vi "Load config.vi"(8 "error in (no error)":errorcluster, 11 "Data Cluster in":T1) -> (0 "error out":errorcluster, 2 "Call config dialog?":bool, 3 "Data Cluster out":T1)   [LabVIEW 2020, in "UI.lvlib"]
uses:
  UI.lvlib
  Module Data--cluster.ctl
  <vilib>/Utility/file.llb/Application Directory.vi
  <vilib>/Utility/config.llb/Read Key (String).vi
  <vilib>/Utility/config.llb/Read Key (Double).vi
  <vilib>/Utility/config.llb/NI_LVConfig.lvlib
  NI_DAQ/Libraries/NI DAQ/NI DAQ.lvlib
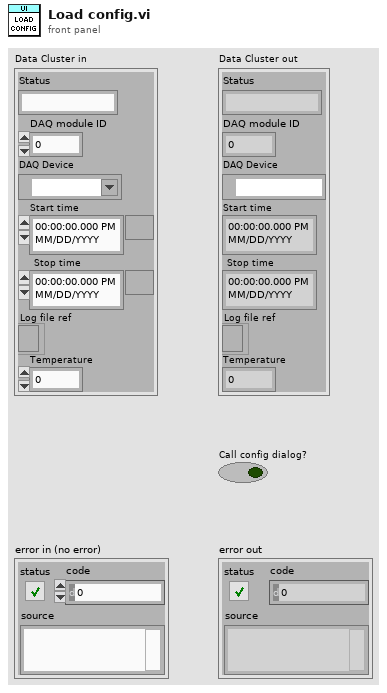
[diagram p1: front panel]
types:
  T1 = typedef "UI.lvlib/Module Data--cluster.ctl" = cluster{"Status":string, "DAQ module ID":i32, "DAQ Device":tag, "Start time":timestamp, "Stop time":timestamp, "Log file ref":refnum<file>, "Temperature":dbl}
  T2 = typedef "NI_LVConfig.lvlib/Config Data RefNum.ctl" = refnum<k1>
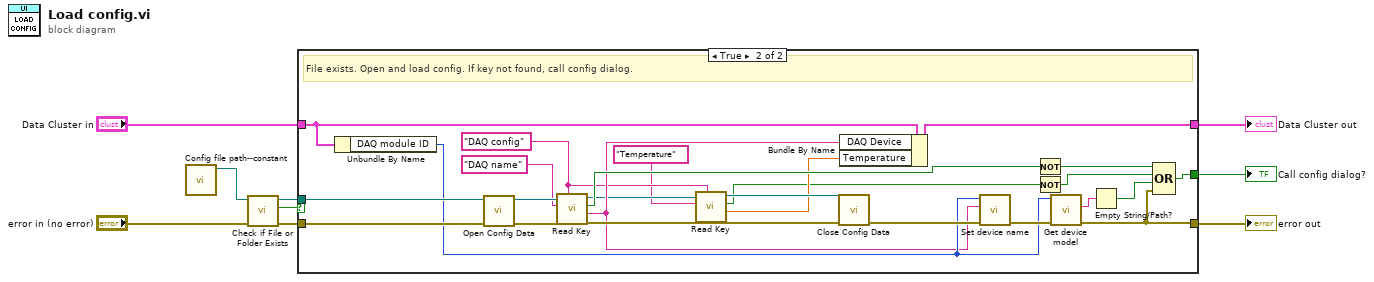
[diagram p0: block diagram]
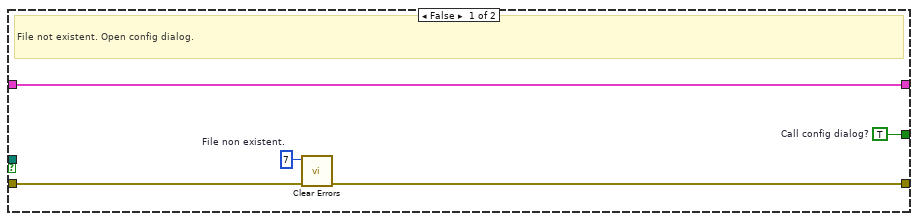
[diagram p2: hidden frame]
diagram:
  n1 = call "Config file path--constant.vi"() -> ("Path"=w3:path)  [unwired: 11 in]
  n2 = call <vilib>:"Check if File or Folder Exists.vi"("error in (no error)"="error in (no error)", "path"=w3) -> ("error out"=w4:errorcluster, "file or folder exists?"=w1:bool, "dup path"=w2:path)  [unwired: 7 in]
  n3 = case shown="True" w1 {
    tunnel: w4 -> [w13 w37]
    tunnel: w2 -> [_ w38]
    tunnel: [w14 w29] -> w9
    tunnel: [w11 w22] -> w6
    tunnel: "Data Cluster in" -> [w12 w30]
    tunnel: [w12 w34] -> w8
    frame False {
      w10 = 7  # File non existent.
      w14 = TRUE  # Call config dialog?
      # "File not existent. Open config dialog."
      n4 = call <vilib>:"Clear Errors.vi"("error in (no error)"=w13, "specific error code to clear (0: all)"=w10) -> ("error out"=w11:errorcluster)  [unwired: 4 in, 1 out]
    }
    frame True {
      w19 = "DAQ config" ("section")
      # "File exists. Open and load config. If key not found, call config dialog."
      n5 = Unbundle By Name(w30) -> ("DAQ module ID"=w24:i32)
      n6 = call <vilib>:"Open Config Data.vi"("error in (no error)"=w37, "configuration file path"=w38) -> ("error out"=w36:errorcluster, "refnum"=w35:T2)  [unwired: 7 in, 1 out]
      n7 = call-poly <vilib>:"Read Key.vi"("section"=w19, "key"="DAQ name", "refnum"=w35) -> ("value"=w23:string, "found?"=w32:bool, "refnum out"=w21:T2)  [unwired: 5 in, 1 out]
      n8 = call-poly <vilib>:"Read Key.vi"("section"=w19, "key"="Temperature", "refnum"=w21) -> ("value"=w17:dbl, "found?"=w16:bool, "refnum out"=w20:T2)  [unwired: 5 in, 1 out]
      n9 = call <vilib>:"Close Config Data.vi"("error in (no error)"=w36, "refnum"=w20) -> ("error out"=w26:errorcluster)  [unwired: 8 in, 1 out]
      n10 = Bundle By Name(cluster=w30, "DAQ Device"=w23, "Temperature"=w17) -> (w34:T1)
      n11 = call "Set device name.vi"("error in"=w26, "Device name"=w23, "Module ID"=w24) -> ("error out"=w25:errorcluster)  [unwired: 8 in]
      n12 = Not(x=w32) -> (.not. x?=w31:bool)
      n13 = Not(x=w16) -> (.not. x?=w15:bool)
      n14 = call "Get device model.vi"("error in"=w25, "Module ID"=w24) -> ("error out"=w22:errorcluster, "Device model"=w28:string)  [unwired: 7 in, 1 out]
      n15 = Empty String/Path?(string/path=w28) -> (empty?=w27:bool)
      n16 = Compound Arithmetic op=OR(w31, w15, w27, w22) -> (w29:bool)
    }
  }
  "Call config dialog?" <- w9
  "Data Cluster out" <- w8
  "error out" <- w6
